vi "database1查询.vi"(7 "终止时间":string, 8 "error in (no error)":errorcluster, 9 "table":string, 10 "起始时间":string, 11 "database":string="database1.mdb") -> (0 "error out":errorcluster, 1 "database溢出":bool, 2 "data":string[][](table), 3 "recordset data":variant[][](array[variant]))   [LabVIEW 2016, in "数据传输系统-04.lvlib"]
uses:
  <vilib>/Utility/sysdir.llb/System Directory Type.ctl
  <vilib>/addons/database/Connection.llb/DB Tools Open Connec (String).vi
  <vilib>/addons/database/Connection.llb/Conn Execute.vi
  <vilib>/addons/database/Recordset.llb/Rec Fetch Recordset Data (R).vi
  <vilib>/addons/database/Recordset.llb/Rec Destroy - Connection.vi
  <vilib>/addons/database/_DB Variant To Data/Database Variant To Data.xnode
  <vilib>/addons/database/NI_Database_API.lvlib
panel:
  out "结果字符串":string
  out "仪器代号":string[](array[string])
  out "连接的字符串":string
  out "SQL query":string
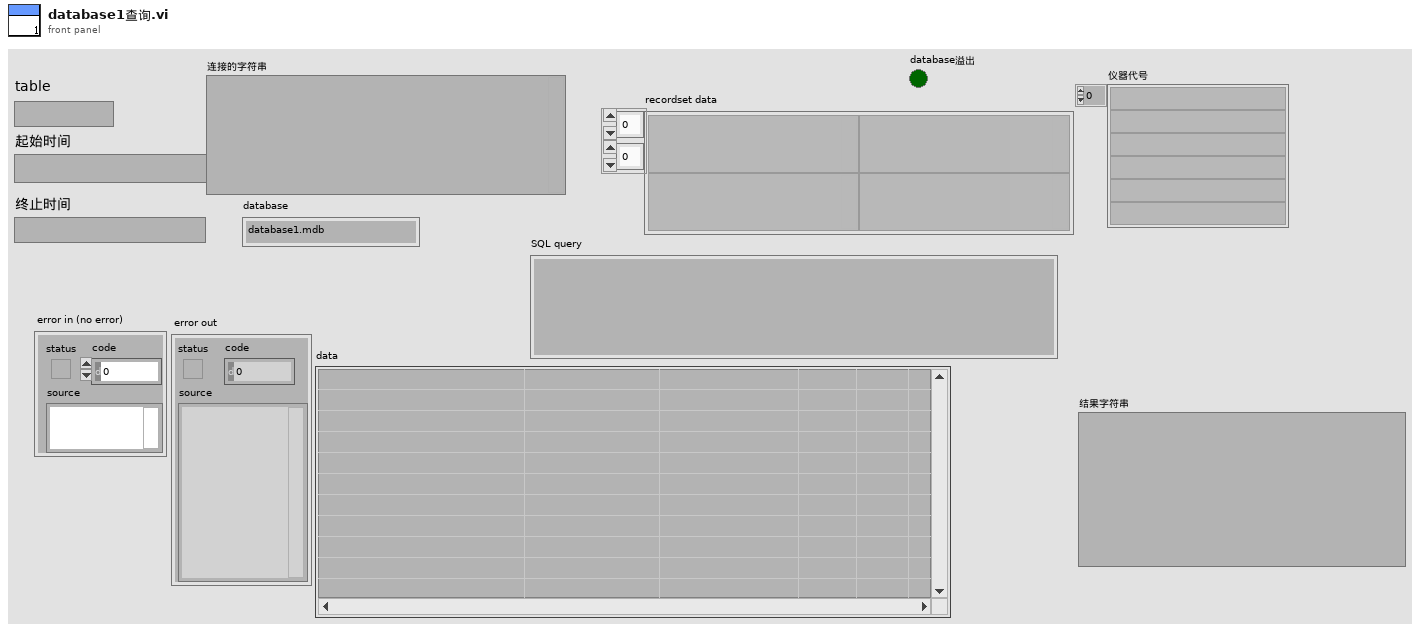
[diagram p1: front panel]
types:
  T1 = typedef "System Directory Type.ctl" = i32
  T2 = typedef "NI_Database_API.lvlib/Conn ObjectReference.ctl" = refnum<k1>
  T3 = typedef "NI_Database_API.lvlib/Rec ObjectReference.ctl" = refnum<k1>
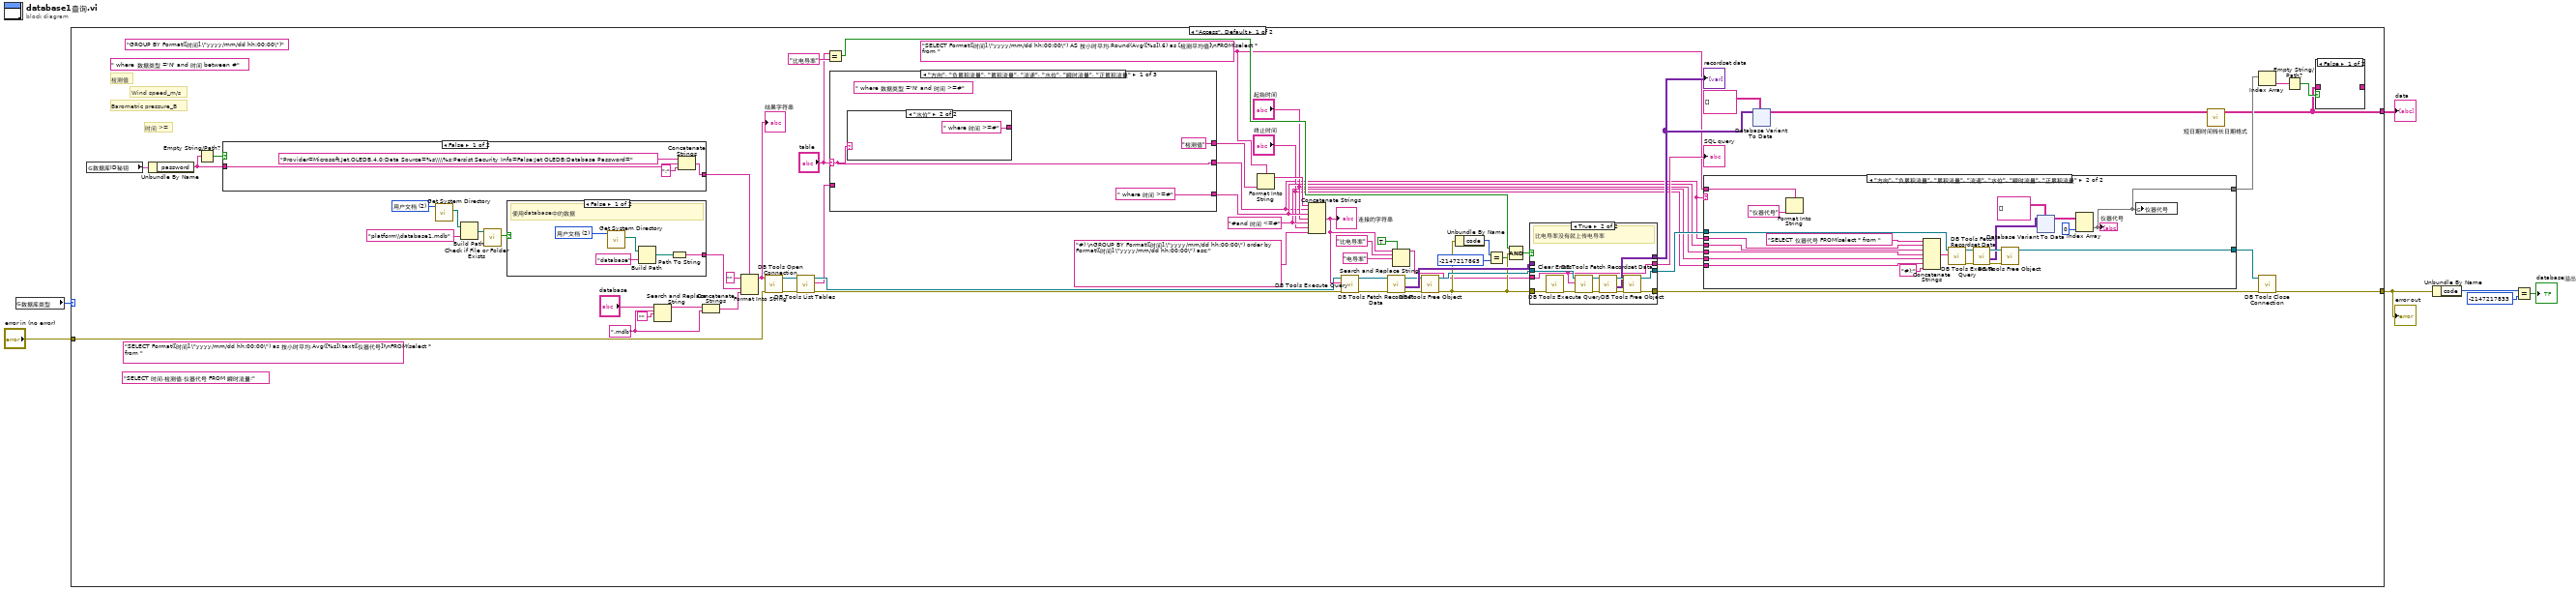
[diagram p0: block diagram]
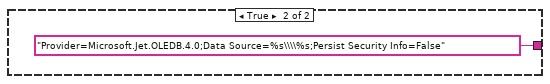
[diagram p4: hidden frame]
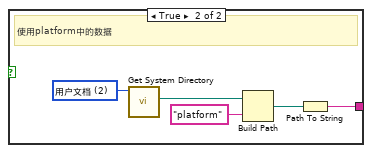
[diagram p6: hidden frame]
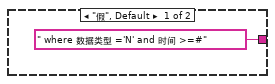
[diagram p7: hidden frame]
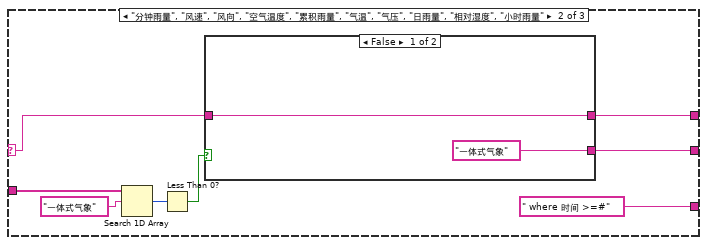
[diagram p8: hidden frame]
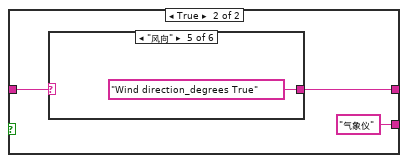
[diagram p9: hidden frame]
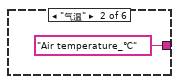
[diagram p11: hidden frame]
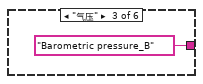
[diagram p12: hidden frame]
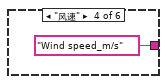
[diagram p13: hidden frame]
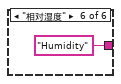
[diagram p14: hidden frame]
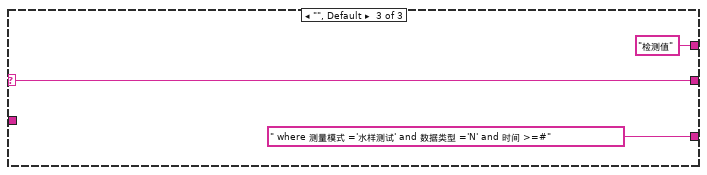
[diagram p15: hidden frame]
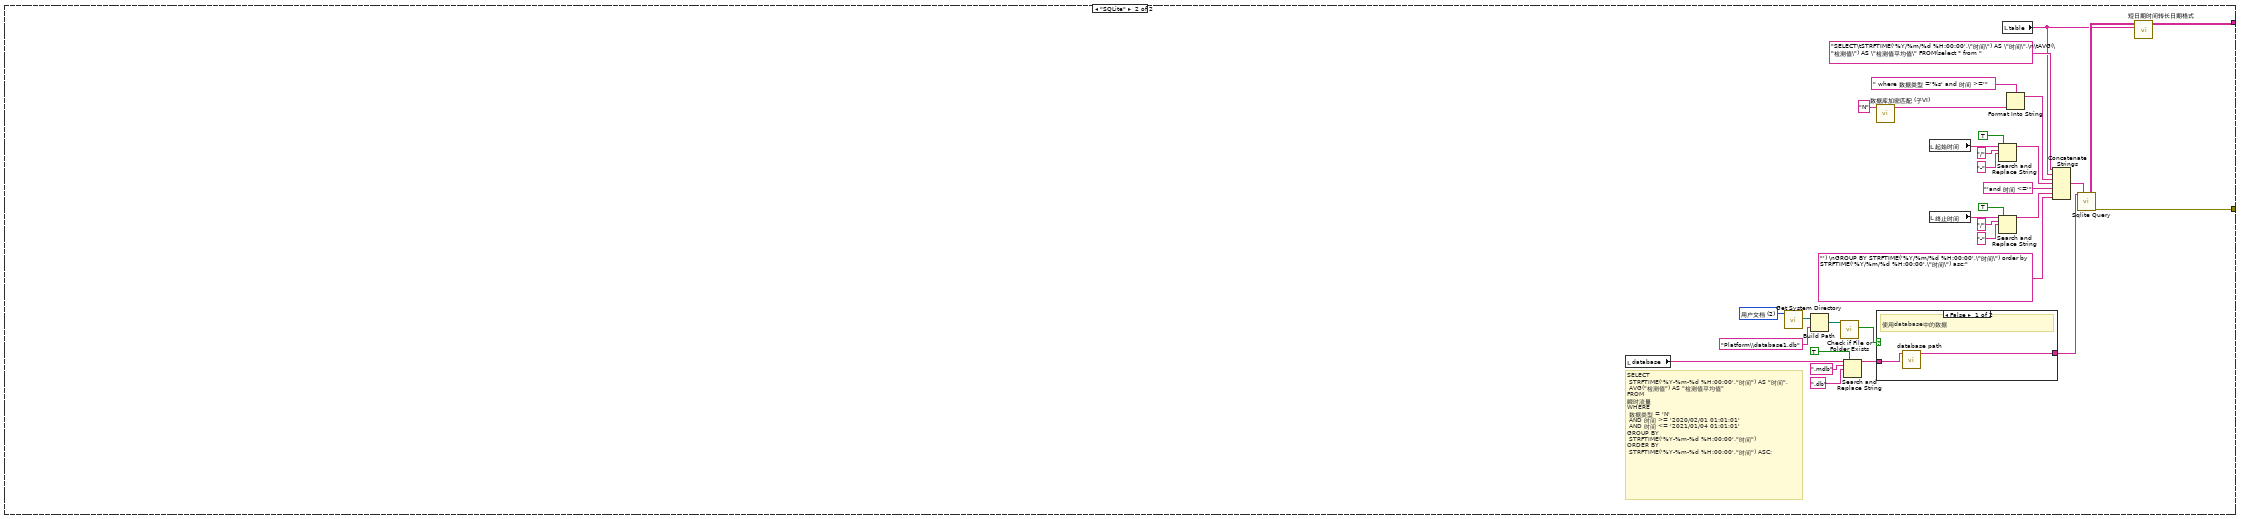
[diagram p16: hidden frame]
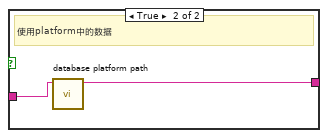
[diagram p17: hidden frame]
diagram:
  n1 = global read "断电保存全局.vi" "数据库类型"() -> (w7:enum16{"Access", "SQLite"})
  n2 = case shown="\"Access\", Default" w7 {
    tunnel: [w38 w248] -> w4
    tunnel: "error in (no error)" -> [w37 _]
    tunnel: [w13 w264] -> w5
    frame "Access", Default {
      w18 = "SELECT Format([时间],\"yyyy/mm/dd hh:00:00\") AS 按小时平均,Round(Avg([%s]),6) as [检测平均值]\nFROM(select * from "
      (unwired) "SELECT 时间,检测值,仪器代号 FROM 瞬时流量;" ("连接的字符串")
      w30 = ".mdb" ("搜索字符串")
      (unwired) " where 数据类型 ='N' and 时间 between #"
      w67 = T1 2 items=["用户目录"=0, "用户桌面"=1, "用户文档"=2, "用户应用程序数据"=3, "用户设置"=4, "用户临时目录"=5, "公共文档"=6, "公共应用程序数据"=7, "公共设置"=8, "公共缓存"=13, "系统核心库"=9, "系统安装库"=10, "应用程序文件"=11, "启动盘根目录"=12] ("system directory type")
      (unwired) "GROUP BY Format([时间],\"yyyy/mm/dd hh:00:00\")"
      w23 = "#and 时间 <=#"
      (unwired) "SELECT Format([时间],\"yyyy/mm/dd hh:00:00\") as 按小时平均,Avg([%s]),text([仪器代号])\nFROM(select * from "
      # "时间 >="
      # "Wind speed_m/s"
      # "检测值"
      # "Barometric pressure_B"
      n3 = global read "外部交互全局.vi" "数据库ID秘钥"() -> (w39:cluster{"userID":string, "password":string})
      n4 = Unbundle By Name(w39) -> ("password"=w41:string)
      n5 = Empty String/Path?(string/path=w41) -> (empty?=w14:bool)
      n6 = case shown="False" w14 {
        tunnel: [w183 "Provider=Microsoft.Jet.OLEDB.4.0;Data Source=%s\\\\%s;Persist Security Info=False" ("格式字符串")] -> w40
        tunnel: w41 -> [w182 _]
        frame False {
          n7 = Concatenate Strings("Provider=Microsoft.Jet.OLEDB.4.0;Data Source=%s\\\\%s;Persist Security Info=False;Jet OLEDB:Database Password=" ("格式字符串"), w182, ";" ("字符串")) -> (w183:string)
        }
        frame True {
        }
      }
      n8 = call <vilib>:"Get System Directory.vi"("system directory type"=w67) -> ("system directory"=w68:path)  [unwired: 10 in]
      n9 = Build Path(base path=w68, name or relative path="platform\\database1.mdb" ("condition")) -> (appended path=w66:path)
      n10 = call <vilib>:"Check if File or Folder Exists.vi"("path"=w66) -> ("file or folder exists?"=w64:bool)  [unwired: 8 in, 2 out]
      n11 = case shown="False" w64 {
        tunnel: [w202 w207] -> w63
        frame False {
          w205 = T1 2 items=["用户目录"=0, "用户桌面"=1, "用户文档"=2, "用户应用程序数据"=3, "用户设置"=4, "用户临时目录"=5, "公共文档"=6, "公共应用程序数据"=7, "公共设置"=8, "公共缓存"=13, "系统核心库"=9, "系统安装库"=10, "应用程序文件"=11, "启动盘根目录"=12] ("system directory type")
          # "使用database中的数据"
          n12 = call <vilib>:"Get System Directory.vi"("system directory type"=w205) -> ("system directory"=w204:path)  [unwired: 10 in]
          n13 = Build Path(base path=w204, name or relative path="database" ("condition")) -> (appended path=w206:path)
          n14 = Path To String(path=w206) -> (string=w202:string)
        }
        frame True {
          w211 = T1 2 items=["用户目录"=0, "用户桌面"=1, "用户文档"=2, "用户应用程序数据"=3, "用户设置"=4, "用户临时目录"=5, "公共文档"=6, "公共应用程序数据"=7, "公共设置"=8, "公共缓存"=13, "系统核心库"=9, "系统安装库"=10, "应用程序文件"=11, "启动盘根目录"=12] ("system directory type")
          # "使用platform中的数据"
          n15 = call <vilib>:"Get System Directory.vi"("system directory type"=w211) -> ("system directory"=w210:path)  [unwired: 10 in]
          n16 = Build Path(base path=w210, name or relative path="platform" ("condition")) -> (appended path=w208:path)
          n17 = Path To String(path=w208) -> (string=w207:string)
        }
      }
      n18 = Search and Replace String(input string="database", search string=w30, replace string="") -> (result string=w31:string)  [unwired: 5 in, 3 out]
      n19 = Concatenate Strings(w31, w30) -> (w28:string)
      n20 = Format Into String(format string=w40, initial string="" ("初始字符串"), w63, w28) -> (resulting string=w62:string)  [unwired: 1 in, 1 out]
      "结果字符串" <- w62
      n21 = call-poly <vilib>:"DB Tools Open Connection.vi"("error in (no error)"=w37, "connection information"=w62) -> ("error out"=w12:errorcluster, "connection reference"=w11:T2)  [unwired: 6 in]
      n22 = call <vilib>:"DB Tools List Tables.vi"("error in (no error)"=w12, "connection reference"=w11) -> ("error out"=w9:errorcluster, "tables"=w8:string[], "connection reference out"=w10:T2)  [unwired: 3 in]
      n23 = Equal?(x="table", y="比电导率") -> (x = y?=w57:bool)
      n24 = case shown="\"方向\", \"负累积流量\", \"累积流量\", \"流速\", \"水位\", \"瞬时流量\", \"正累积流量\"" "table" {
        selector: "table" -> [w213 w218 w237]
        tunnel: [" where 时间 >=#" " where 时间 >=#" " where 测量模式 ='水样测试' and 数据类型 ='N' and 时间 >=#"] -> w25
        tunnel: ["检测值" w217 "检测值"] -> w44
        tunnel: [w213 w223 w237] -> w20
        tunnel: w8 -> [_ w222 _]
        frame "方向", "负累积流量", "累积流量", "流速", "水位", "瞬时流量", "正累积流量" {
          (unwired) " where 数据类型 ='N' and 时间 >=#"
          n25 = case shown="\"水位\"" w213 {
            tunnel: [" where 数据类型 ='N' and 时间 >=#" " where 时间 >=#"] -> _
            frame "假", Default {
            }
            frame "水位" {
            }
          }
        }
        frame "分钟雨量", "风速", "风向", "空气温度", "累积雨量", "气温", "气压", "日雨量", "相对湿度", "小时雨量" {
          n26 = Search 1D Array(1D array=w222, element="一体式气象") -> (index of element=w220:i32)  [unwired: 1 in]
          n27 = Less Than 0?(x=w220) -> (x < 0?=w219:bool)
          n28 = case shown="False" w219 {
            tunnel: ["一体式气象" "气象仪"] -> w223
            tunnel: w218 -> [w225 w229]
            tunnel: [w225 w227] -> w217
            frame False {
            }
            frame True {
              n29 = case shown="\"风向\"" w229 {
                selector: w229 -> [w230 _ _ _ _ _]
                tunnel: [w230 "Air temperature_℃" "Barometric pressure_B" "Wind speed_m/s" "Wind direction_degrees True" "Humidity"] -> w227
                frame Default {
                }
                frame "气温" {
                }
                frame "气压" {
                }
                frame "风速" {
                }
                frame "风向" {
                }
                frame "相对湿度" {
                }
              }
            }
          }
        }
        frame "", Default {
        }
      }
      n30 = Format Into String(format string=w18, w44) -> (resulting string=w42:string)  [unwired: 2 in, 1 out]
      n31 = Concatenate Strings(w42, w20, w25, "起始时间", w23, "终止时间", "#) \nGROUP BY Format([时间],\"yyyy/mm/dd hh:00:00\") order by Format([时间],\"yyyy/mm/dd hh:00:00\") asc;" ("字符串")) -> (w27:string)
      "连接的字符串" <- w27
      n32 = call-poly <vilib>:"DB Tools Execute Query.vi"("error in (no error)"=w9, "SQL query"=w27, "connection reference"=w10) -> ("error out"=w55:errorcluster, "recordset reference"=w59:T3)  [unwired: 5 in]
      n33 = call-poly <vilib>:"DB Tools Fetch Recordset Data.vi"("error in (no error)"=w55, "recordset reference"=w59) -> ("error out"=w70:errorcluster, "recordset data"=w60:variant[][], "recordset reference out"=w56:T3)  [unwired: 3 in]
      n34 = Search and Replace String(replace all?=TRUE ("替换全部？(F)"), input string=w27, search string="比电导率" ("搜索字符串"), replace string="电导率" ("替换字符串(\"\")")) -> (result string=w47:string)  [unwired: 4 in, 3 out]
      n35 = call-poly <vilib>:"DB Tools Free Object.vi"("error in (no error)"=w70, "recordset reference"=w56) -> ("error out"=w51:errorcluster, "connection reference"=w54:T2)  [unwired: 8 in]
      n36 = Unbundle By Name(w51) -> ("code"=w53:i32)
      n37 = Equal?(x=w53, y=-2147217865 ("code")) -> (x = y?=w50:bool)
      n38 = Compound Arithmetic op=AND ("复合运算")(w57, w51, w50) -> (w61:bool)
      n39 = case shown="True" w61 {
        tunnel: w47 -> [w187 w191]
        tunnel: w54 -> [w188 w196]
        tunnel: [w188 w192] -> w26
        tunnel: [w190 w194] -> w33
        tunnel: w60 -> [w190 _]
        tunnel: w51 -> [w189 w201]
        tunnel: [w189 w193] -> w34
        tunnel: [w187 w191] -> w45
        frame False {
        }
        frame True {
          # "比电导率没有就上传电导率"
          n40 = call <vilib>:"Clear Errors.vi"("error in (no error)"=w201) -> ("error out"=w195:errorcluster)  [unwired: 5 in, 1 out]
          n41 = call-poly <vilib>:"DB Tools Execute Query.vi"("error in (no error)"=w195, "SQL query"=w191, "connection reference"=w196) -> ("error out"=w197:errorcluster, "recordset reference"=w199:T3)  [unwired: 5 in]
          n42 = call-poly <vilib>:"DB Tools Fetch Recordset Data.vi"("error in (no error)"=w197, "recordset reference"=w199) -> ("error out"=w200:errorcluster, "recordset data"=w194:variant[][], "recordset reference out"=w198:T3)  [unwired: 3 in]
          n43 = call-poly <vilib>:"DB Tools Free Object.vi"("error in (no error)"=w200, "recordset reference"=w198) -> ("error out"=w193:errorcluster, "connection reference"=w192:T2)  [unwired: 8 in]
        }
      }
      "SQL query" <- w45
      "recordset data" <- w33
      n44 = case shown="\"方向\", \"负累积流量\", \"累积流量\", \"流速\", \"水位\", \"瞬时流量\", \"正累积流量\"" w20 {
        tunnel: w26 -> [w72 w89]
        tunnel: w20 -> [_ w88]
        tunnel: w25 -> [_ w87]
        tunnel: "起始时间" -> [_ w86]
        tunnel: w23 -> [_ w85]
        tunnel: "终止时间" -> [_ w84]
        tunnel: [w72 w81] -> w21
        tunnel: w18 -> [_ w76]
        tunnel: [_ w73] -> w17
        frame "假", Default {
        }
        frame "方向", "负累积流量", "累积流量", "流速", "水位", "瞬时流量", "正累积流量" {
          n45 = Format Into String(format string=w76, "仪器代号" ("输入 1")) -> ()  [unwired: 2 in, 2 out]
          n46 = Concatenate Strings("SELECT 仪器代号 FROM(select * from " ("连接的字符串"), w88, w87, w86, w85, w84, "#);" ("连接的字符串")) -> (w82:string)
          n47 = call-poly <vilib>:"DB Tools Execute Query.vi"("SQL query"=w82, "connection reference"=w89) -> ("error out"=w93:errorcluster, "recordset reference"=w91:T3)  [unwired: 6 in]
          n48 = call-poly <vilib>:"DB Tools Fetch Recordset Data.vi"("error in (no error)"=w93, "recordset reference"=w91) -> ("error out"=w90:errorcluster, "recordset data"=w80:variant[][], "recordset reference out"=w92:T3)  [unwired: 3 in]
          n49 = call-poly <vilib>:"DB Tools Free Object.vi"("error in (no error)"=w90, "recordset reference"=w92) -> ("connection reference"=w81:T2)  [unwired: 8 in, 1 out]
          n50 = xnode "Database Variant To Data"("database variant"=w80, "type"=string[][] []) -> ("data"=w78:string[][])  [unwired: 1 in, 1 out]
          n51 = Index Array(array=w78, index (col)=0 ("禁用的索引 (列)")) -> (element=w73:string[])  [unwired: 1 in]
          "仪器代号" <- w73
          n52 = global write "全局 所有参数.vi" "仪器代号"(w73) -> ()
        }
      }
      n53 = xnode "Database Variant To Data"("database variant"=w33, "type"=string[][] []) -> ("data"=w35:string[][])  [unwired: 1 in, 1 out]
      n54 = call "短日期时间转长日期格式.vi"("data"=w35) -> ("输出数组"=w13:string[][])  [unwired: 10 in]
      n55 = Index Array(array=w17) -> (element=w16:string)  [unwired: 1 in]
      n56 = call <vilib>:"DB Tools Close Connection.vi"("error in (no error)"=w34, "connection reference"=w21) -> ("error out"=w38:errorcluster)  [unwired: 5 in]
      n57 = Empty String/Path?(string/path=w16) -> (empty?=w15:bool)
      n58 = case shown="False" w15 {
        tunnel: w13 -> [_ w71]
        tunnel: [_ w71] -> _
        frame False {
        }
        frame True {
        }
      }
    }
    frame "SQLite" {
      w268 = T1 2 items=["用户目录"=0, "用户桌面"=1, "用户文档"=2, "用户应用程序数据"=3, "用户设置"=4, "用户临时目录"=5, "公共文档"=6, "公共应用程序数据"=7, "公共设置"=8, "公共缓存"=13, "系统核心库"=9, "系统安装库"=10, "应用程序文件"=11, "启动盘根目录"=12] ("system directory type")
      # "SELECT\n\tSTRFTIME('%Y-%m-%d %H:00:00',\"时间\") AS \"时间\",\n\tAVG(\"检测值\") AS \"检测值平均值\"\nFROM\n瞬时流量 \nWHERE\n\t数据类型 = 'N' \n\tAND 时间 >= '2020/02/01 01:01:01' \n\tAND 时间 <= '2021/01/04 01:01:01' \nGROUP BY\n\tSTRFTIME('%Y-%m-%d %H:00:00',\"时间\")\nORDER BY\n\tSTRFTIME('%Y-%m-%d %H:00:00',\"时间\") ASC;"
      n59 = local read "database"() -> (w249:string)
      n60 = call <vilib>:"Get System Directory.vi"("system directory type"=w268) -> ("system directory"=w267:path)  [unwired: 10 in]
      n61 = Build Path(base path=w267, name or relative path="Platform\\database1.db" ("condition")) -> (appended path=w269:path)
      n62 = call <vilib>:"Check if File or Folder Exists.vi"("path"=w269) -> ("file or folder exists?"=w271:bool)  [unwired: 8 in, 2 out]
      n63 = Search and Replace String(replace all?=TRUE ("替换全部？(F)"), input string=w249, search string=".mdb" ("搜索字符串"), replace string=".db" ("替换字符串(\"\")")) -> (result string=w240:string)  [unwired: 4 in, 3 out]
      n64 = call "数据库加密匹配 (子VI).vi"("输入参数"="N") -> ("Encoded String"=w242:string)  [unwired: 10 in]
      n65 = case shown="False" w271 {
        tunnel: [w272 w274] -> w239
        tunnel: w240 -> [w273 w275]
        frame False {
          # "使用database中的数据"
          n66 = call "database path.vi"("database"=w273) -> ("Path out"=w272:string)  [unwired: 9 in, 1 out]
        }
        frame True {
          # "使用platform中的数据"
          n67 = call "database platform path.vi"("database"=w275) -> ("Path out"=w274:string)  [unwired: 10 in]
        }
      }
      n68 = local read "起始时间"() -> (w256:string)
      n69 = local read "终止时间"() -> (w254:string)
      n70 = Search and Replace String(replace all?=TRUE ("替换全部？(F)"), input string=w256, search string="/" ("搜索字符串"), replace string="-" ("替换字符串(\"\")")) -> (result string=w255:string)  [unwired: 4 in, 3 out]
      n71 = Search and Replace String(replace all?=TRUE ("替换全部？(F)"), input string=w254, search string="/" ("搜索字符串"), replace string="-" ("替换字符串(\"\")")) -> (result string=w253:string)  [unwired: 4 in, 3 out]
      n72 = local read "table"() -> (w246:string)
      n73 = Format Into String(format string=" where 数据类型 ='%s' and 时间 >='", w242) -> (resulting string=w244:string)  [unwired: 2 in, 1 out]
      n74 = Concatenate Strings("SELECT\tSTRFTIME('%Y/%m/%d %H:00:00',\"时间\") AS \"时间\",\n\tAVG(\"检测值\") AS \"检测值平均值\" FROM(select * from ", w246, w244, w255, "'and 时间 <='", w253, "') \nGROUP BY STRFTIME('%Y/%m/%d %H:00:00',\"时间\") order by STRFTIME('%Y/%m/%d %H:00:00',\"时间\") asc;" ("字符串")) -> (w241:string)
      n75 = call "Sqlite Query.vi"("DB Path"=w239, "SQL Query"=w241) -> ("Results"=w247:string[][], "error out"=w248:errorcluster)  [unwired: 11 in, 1 out]
      n76 = call "短日期时间转长日期格式.vi"("table输入"=w246, "data"=w247) -> ("输出数组"=w264:string[][])  [unwired: 9 in]
    }
  }
  "error out" <- w4
  "data" <- w5
  n77 = Unbundle By Name(w4) -> ("code"=w3:i32)
  n78 = Equal?(x=w3, y=-2147217833 ("code")) -> (x = y?=→"database溢出":bool)
